vi "End.vi"(8 "error in (no error)":errorcluster, 11 "Simulated_CCD_Camera in":refnum<class "Simulated Camera.lvclass">) -> (0 "error out":errorcluster, 3 "Simulated_CCD_Camera out":refnum<class "Simulated Camera.lvclass">)   [LabVIEW 2018, in "Simulated Camera.lvclass"]
doc: "Correctly ends communication with the camera."
uses:
  Simulated Camera.lvclass
  Simulated Camera.lvclass/Simulated Camera.ctl
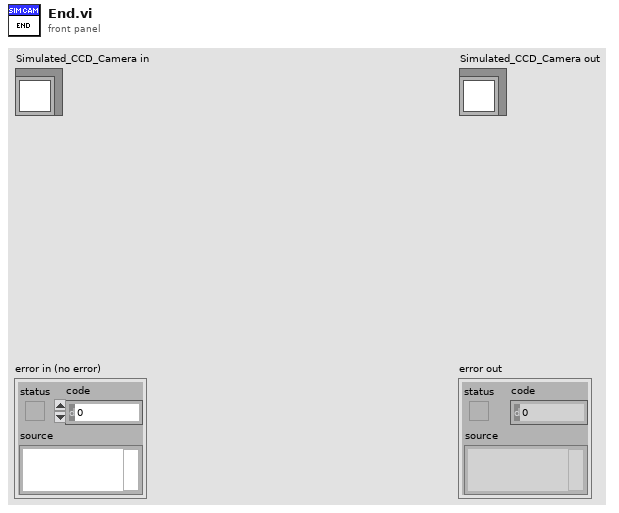
[diagram p1: front panel]
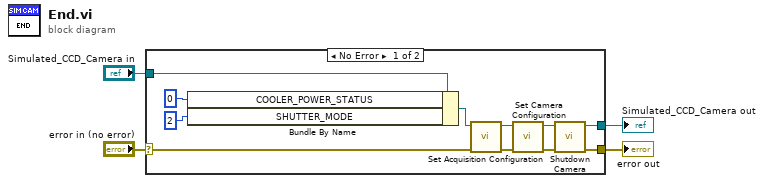
[diagram p0: block diagram]
diagram:
  n1 = case shown="No Error" "error in (no error)" {
    selector: "error in (no error)" -> [w9 w17]
    tunnel: [w14 w17] -> w3
    tunnel: [w13 w16] -> w1
    tunnel: "Simulated_CCD_Camera in" -> [w12 w16]
    frame No Error {
      n2 = Bundle By Name(cluster=w12, "COOLER_POWER_STATUS"=u16 0, "SHUTTER_MODE"=u16 2 ("New CCD Config.SHUTTER_MODE")) -> (w10:refnum<class "Simulated Camera.lvclass">)
      n3 = call-dynamic "Set Acquisition Configuration.vi"("error in (no error)"=w9, "CCDCamera in"=w10) -> ("error out"=w5:errorcluster, "CCDCamera out"=w8:refnum<class "Simulated Camera.lvclass">)  [unwired: 8 in]
      n4 = call-dynamic "Set Camera Configuration.vi"("error in (no error)"=w5, "CCDCamera in"=w8) -> ("error out"=w6:errorcluster, "CCDCamera out"=w7:refnum<class "Simulated Camera.lvclass">)  [unwired: 8 in]
      n5 = call-dynamic "Shutdown Camera.vi"("error in (no error)"=w6, "CCDCamera in"=w7) -> ("error out"=w14:errorcluster, "CCDCamera out"=w13:refnum<class "Simulated Camera.lvclass">)  [unwired: 8 in]
    }
    frame Error {
    }
  }
  "error out" <- w3
  "Simulated_CCD_Camera out" <- w1
